vi "Read XY 7265.vi"(8 "error in (no error)":errorcluster, 11 "7265 GPIB":string="7") -> (0 "error out":errorcluster, 2 "Y channel":dbl=0.00012, 3 "X channel":dbl=0.009985)   [LabVIEW 2014]
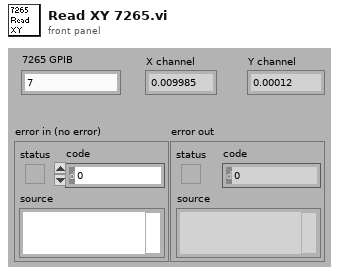
[diagram p1: front panel]
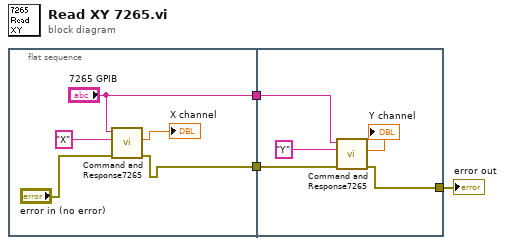
[diagram p0: block diagram]
diagram:
  n1 = flat-sequence {
    tunnel: ["7265 GPIB"] -> w3
    tunnel: [w4] -> w2
    tunnel: w3 -> [w13]
    tunnel: w2 -> [w11]
    tunnel: [w9] -> w1
    frame #0 {
      n2 = call "Command and Response7265.vi"("error in (no error)"="error in (no error)", "Command"="X", "7265 GPIB"="7265 GPIB") -> ("error out"=w4:errorcluster, "Response Code Only"=→"X channel":dbl)  [unwired: 6 in, 1 out]
    }
    frame #1 {
      n3 = call "Command and Response7265.vi"("error in (no error)"=w11, "Command"="Y", "7265 GPIB"=w13) -> ("error out"=w9:errorcluster, "Response Code Only"=→"Y channel":dbl)  [unwired: 6 in, 1 out]
    }
  }
  "error out" <- w1
